vi "FTW-Router-Worker-Launch.vi"(0 "Message Handler":refnum<user-event>, 5 "FTW-Endpoint in":refnum<class "FTW-Endpoint.lvclass">, 11 "error in":errorcluster) -> (15 "error out":errorcluster)   [LabVIEW 2013, in "FTW-Router.lvclass"]
uses:
  FTW-Router.lvclass
  Endpoint/FTW-Endpoint.lvclass
  Message/Request/FTW-Message-IncomingRequest.lvclass
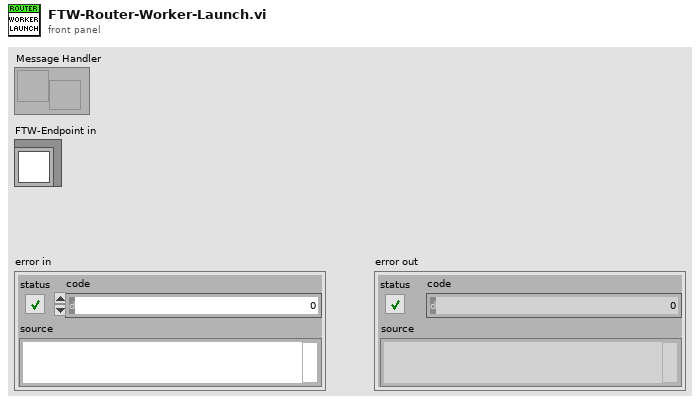
[diagram p1: front panel]
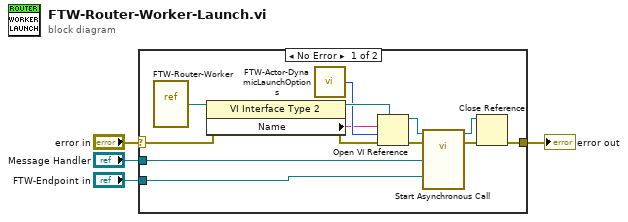
[diagram p0: block diagram]
diagram:
  n1 = case shown="No Error" "error in" {
    selector: "error in" -> [w6 w18]
    tunnel: "FTW-Endpoint in" -> [w16 _]
    tunnel: "Message Handler" -> [w15 _]
    tunnel: [w5 w18] -> w1
    frame No Error {
      n2 = vi-ref "FTW-Router-Worker.vi"() -> (w7:refnum<vi>)
      n3 = property class="VI Interface Type 2"(reference=w7, error in=w6) -> (reference out=w13:refnum<vi>, error out=w8:errorcluster, "Name"=w9:string)
      n4 = call "FTW-Actor-DynamicLaunchOptions.vi"() -> ("Open VI Ref Options"=w10:i32)
      n5 = Open VI Reference(type specifier VI Refnum (for type only)=w13, vi path=w9, options=w10, error in (no error)=w8) -> (vi reference=w12:refnum<vi>, error out=w11:errorcluster)  [unwired: 2 in]
      n6 = call-by-ref "Start Asynchronous Call"(reference=w12, error in=w11, "Endpoint"=w16, "Message Handler"=w15) -> (reference out=w17:refnum<vi>, error out=w14:errorcluster)  [unwired: 1 in]
      n7 = Close Reference(reference=w17, error in (no error)=w14) -> (error out=w5:errorcluster)
    }
    frame Error {
    }
  }
  "error out" <- w1
